vi "Grids.vi"(4 "Properties":T1={"Line"={"Style"=enum."Automatic", "Color"=2147483647, "Width"=nan}} {"Line"."Color" items=["Automatic"=2147483647, "Black"=0, "White"=16777215, "Red"=16711680, "Green"=2263842, "Blue"=255, "Cyan"=65535, "Magenta"=16711935, "Yellow"=16776960]}, 8 "error in (no error)":errorcluster, 9 "Y Grid Lines (T)":bool=TRUE, 10 "X Grid Lines (T)":bool=TRUE, 11 "Plot ID":T5 format="%x") -> (0 "error out":errorcluster, 3 "Plot ID Out":T5 format="%x")   [LabVIEW 2013, in "Advanced Plotting Toolkit.lvlib"]
doc: "Show or hide grid lines. Lines originate at X and Y tick locations."
uses:
  Advanced Plotting Toolkit.lvlib
  typedefs/PlotID.ctl
  GridsProperties.ctl
  properties/Line.ctl
  properties/Line_Style.ctl
  typedefs/PlotColor.ctl
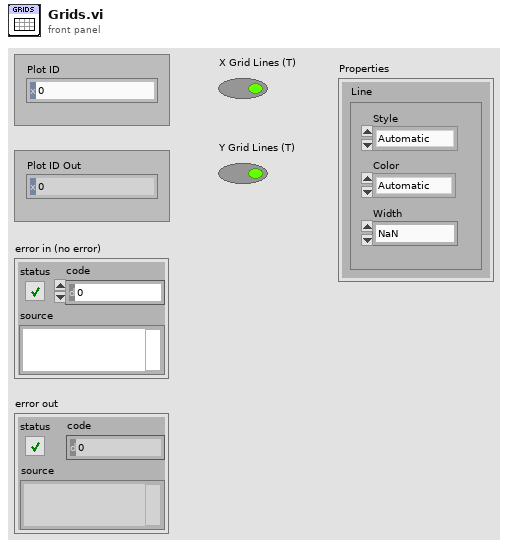
[diagram p1: front panel]
types:
  T1 = typedef "Advanced Plotting Toolkit.lvlib/GridsProperties.ctl" = cluster{"Line":T2}
  T2 = typedef "Advanced Plotting Toolkit.lvlib/Line.ctl" = cluster{"Style":T3, "Color":T4, "Width":sgl}
  T3 = typedef "Advanced Plotting Toolkit.lvlib/Line_Style.ctl" = enum16{"Automatic", "Solid", "Dashed", "Dotted", "Dash-dot", "Invisible"}
  T4 = typedef "Advanced Plotting Toolkit.lvlib/PlotColor.ctl" = u32
  T5 = typedef "Advanced Plotting Toolkit.lvlib/PlotID.ctl" = i32
  T6 = typedef "Advanced Plotting Toolkit.lvlib/KeyValue.ctl" = cluster{"Key":string, "Value":string}
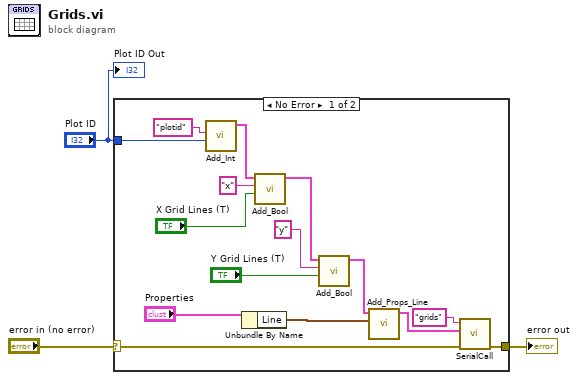
[diagram p0: block diagram]
diagram:
  n1 = case shown="No Error" "error in (no error)" {
    selector: "error in (no error)" -> [w16 w19]
    tunnel: "Plot ID" -> [w18 _]
    tunnel: [w15 w19] -> w1
    frame No Error {
      n2 = call "Add_Int.vi"("Value"=w18, "Key"="plotid") -> ("Keyword Array Out"=w10:T6[])  [unwired: 9 in]
      n3 = Unbundle By Name("Properties") -> ("Line"=w4:T2)
      n4 = call "Add_Bool.vi"("Value"="X Grid Lines (T)", "Key"="x", "Keyword Array"=w10) -> ("Keyword Array Out"=w9:T6[])  [unwired: 8 in]
      n5 = call "Add_Bool.vi"("Value"="Y Grid Lines (T)", "Key"="y", "Keyword Array"=w9) -> ("Keyword Array Out"=w8:T6[])  [unwired: 8 in]
      n6 = call "Add_Props_Line.vi"("Line"=w4, "Keyword Array"=w8) -> ("Keyword Array Out"=w7:T6[])  [unwired: 9 in]
      n7 = call "SerialCall.vi"("error in (no error)"=w16, "data"=w7, "Resource"="grids") -> ("error out"=w15:errorcluster)  [unwired: 7 in, 1 out]
    }
    frame Error {
    }
  }
  "error out" <- w1
  "Plot ID Out" <- "Plot ID"
